vi "Single Write.vi"(8 "error in":errorcluster, 9 "portBit":i32=-1, 10 "data":u8, 11 "task in":i32) -> (0 "error out":errorcluster, 3 "task out":i32)   [LabVIEW 2023, in "DO_Relay.lvlib"]
uses:
  DO_Relay.lvlib
  <userlib>/DAQNavi Polymorphic VI/write/DAQNavi Write (Digital U8 1Chan 1Samp).vi
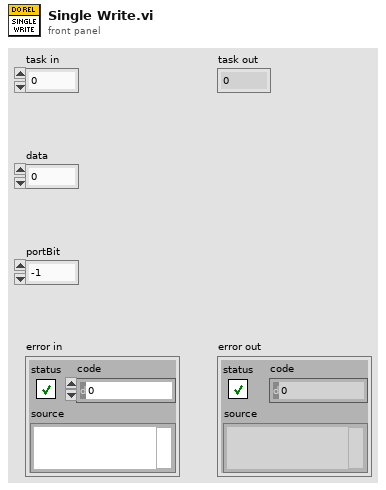
[diagram p1: front panel]
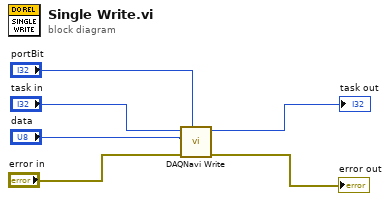
[diagram p0: block diagram]
diagram:
  n1 = call-poly <userlib>:"DAQNavi Write.vi"("portBit"="portBit", "error in (no error)"="error in", "data"="data", "task in"="task in") -> ("error out"=→"error out":errorcluster, "task out"=→"task out":i32)  [unwired: 1 in, 5 out]
